vi "TA Binding Data to String.vi"(8 "error in (no error)":errorcluster, 10 "TA Binding Data":T1, 11 "Motions in":refnum<class "Motions.lvclass">) -> (0 "error out":errorcluster, 2 "String":string, 3 "Motions out":refnum<class "Motions.lvclass">)   [LabVIEW 2016, in "Hardware.lvlib" / "Motions.lvlib" / "Motions.lvclass"]
uses:
  <userlib>/Common Components/Hardware/Abstract System/Motions/Motions/Motions.lvclass
  <userlib>/Common Components/Hardware/Abstract System/Motions/Motions/TA Binding Data.ctl
  <userlib>/Common Components/Hardware/Abstract System/Motions/Motions/Motions.lvclass/Motions.ctl
  <userlib>/Common Components/Hardware/Abstract Hardware/Hardware.lvclass/Hardware.ctl
  <userlib>/Common Components/Hardware/Abstract Hardware/Read Label.vi
  <userlib>/Common Components/Hardware/Motor/Motor/Motor.lvclass
  C:/Program Files (x86)/National Instruments/LabVIEW 2016/user.lib/Common Components/Hardware/Abstract Hardware/Hardware.lvclass
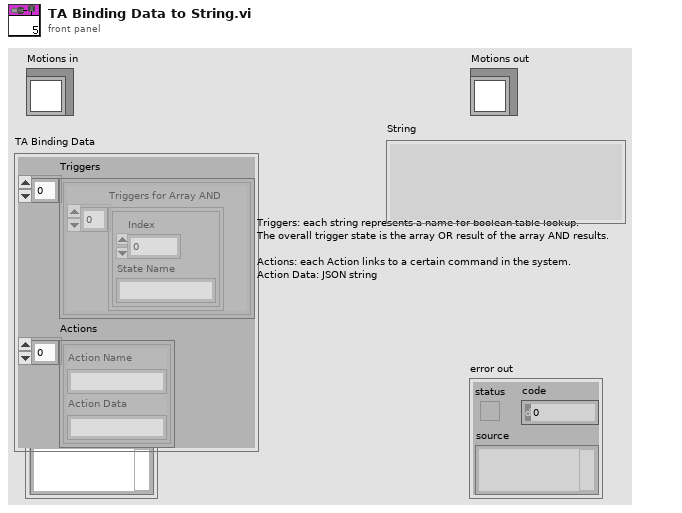
[diagram p1: front panel]
types:
  T1 = typedef "Hardware.lvlib/Motions.lvlib/Motions.lvclass/TA Binding Data.ctl" = cluster{"Triggers":cluster{"Triggers for Array AND":cluster{"Index":u8, "State Name":string}[]}[], "Actions":cluster{"Action Name":string, "Action Data":string}[]}
  T2 = cluster{"Triggers for Array AND":cluster{"Index":u8, "State Name":string}[]}[]
  T3 = cluster{"Action Name":string, "Action Data":string}[]
  T4 = cluster{"Action Name":string, "JSON info":cluster{"path":string, "data type":enum16{"INT", "DBL", "BOOL", "String"}}[], "String Format":string}[]
  T5 = cluster{"path":string, "data type":enum16{"INT", "DBL", "BOOL", "String"}}[]
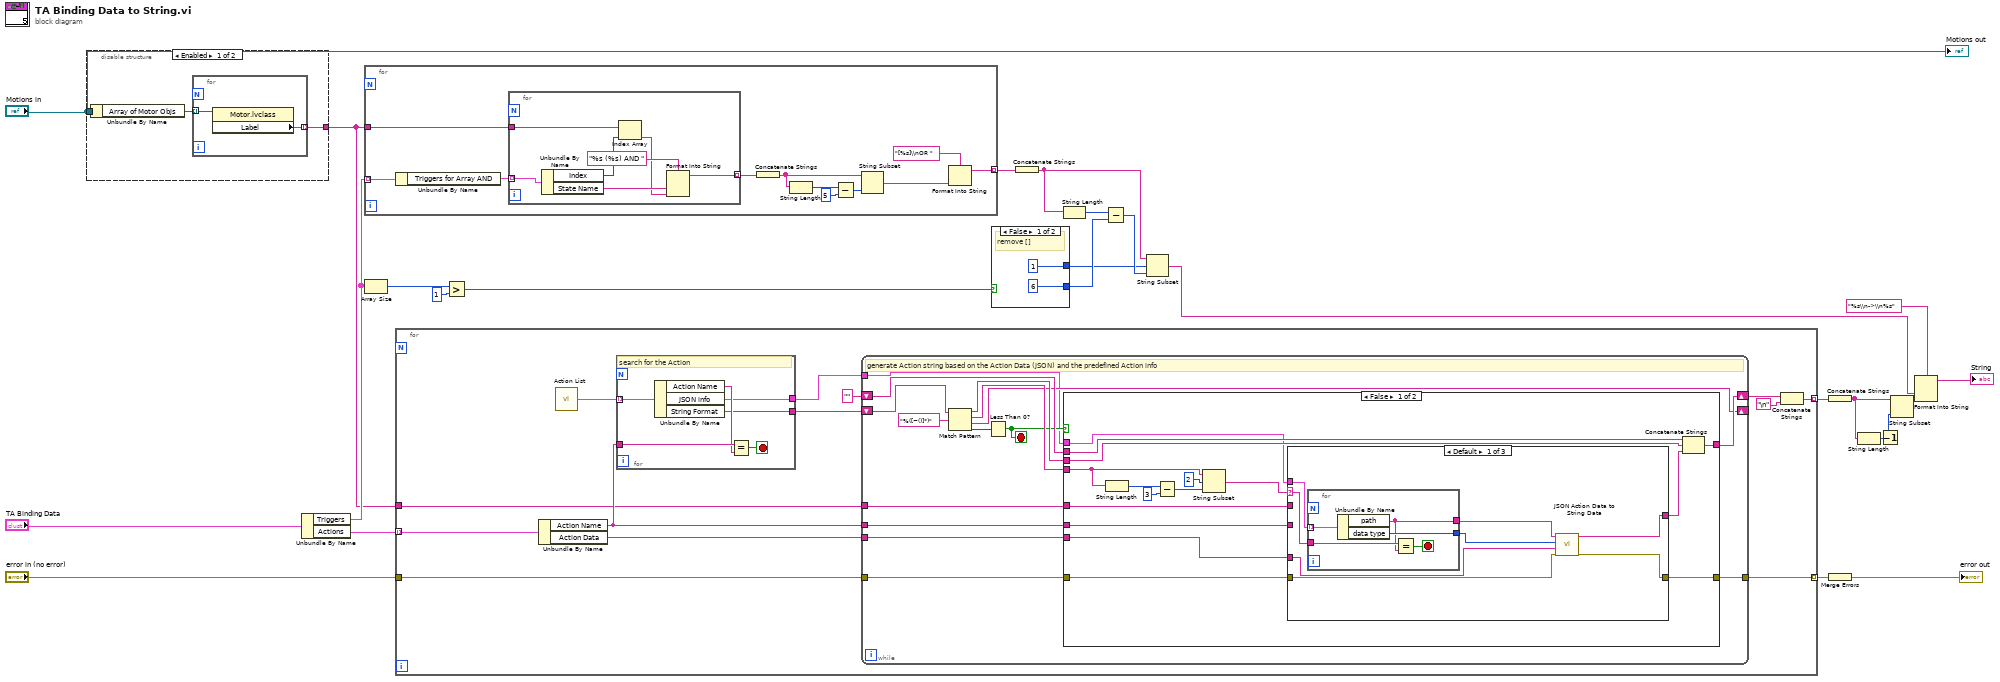
[diagram p0: block diagram]
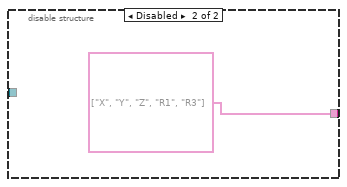
[diagram p2: hidden frame]
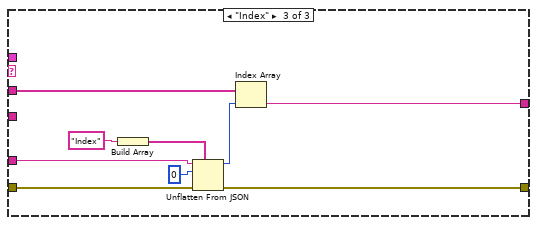
[diagram p4: hidden frame]
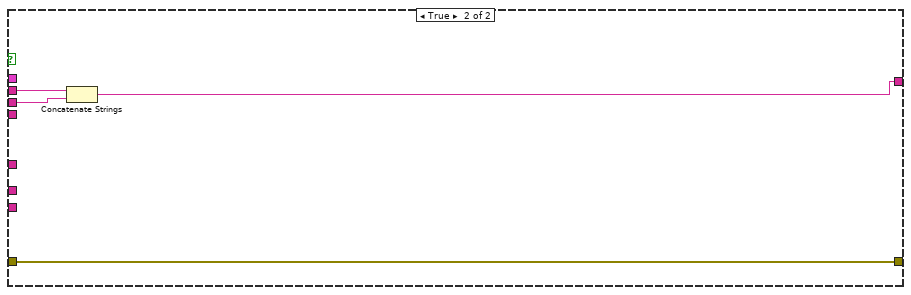
[diagram p5: hidden frame]
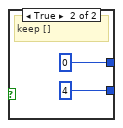
[diagram p6: hidden frame]
diagram:
  n1 = disable-structure shown="Enabled" {
    disable-tunnel: "Motions in" -> [w28 _]
    disable-tunnel: [w26 string[] ["X", "Y", "Z", "R1", "R3"]] -> w9
    frame Enabled {
      n2 = Unbundle By Name(w28) -> ("Array of Motor Objs"=w27:refnum<class "Motor.lvclass">[])
      n3 = for {
        tunnel: w27 -> [w30] mode=indexing
        tunnel: [w29] -> w26 mode=indexing
        n4 = property class="Motor.lvclass"(reference=w30) -> ("Label"=w29:string)  [unwired: 1 in, 2 out]
      }
    }
    frame Disabled {
    }
  }
  n5 = Unbundle By Name("TA Binding Data") -> ("Triggers"=w18:T2, "Actions"=w10:T3)
  n6 = for {
    tunnel: w18 -> [w42] mode=indexing
    tunnel: w9 -> [w40]
    tunnel: [w34] -> w19 mode=indexing
    n7 = Unbundle By Name(w42) -> ("Triggers for Array AND"=w41:cluster{"Index":u8, "State Name":string}[])
    n8 = for {
      tunnel: w41 -> [w49] mode=indexing
      tunnel: w40 -> [w46]
      tunnel: [w43] -> w39 mode=indexing
      n9 = Unbundle By Name(w49) -> ("Index"=w45:u8, "State Name"=w47:string)
      n10 = Index Array(array=w46, index=w45) -> (element=w44:string)
      n11 = Format Into String(format string="%s (%s) AND ", w47, w44) -> (resulting string=w43:string)  [unwired: 2 in, 1 out]
    }
    n12 = Concatenate Strings(w39) -> (w38:string)
    n13 = String Length(string=w38) -> (length=w37:i32)
    n14 = Subtract(x=w37, y=5) -> (x-y=w35:i32)
    n15 = String Subset(string=w38, length (rest)=w35) -> (substring=w32:string)  [unwired: 1 in]
    n16 = Format Into String(format string="[%s]\\nOR ", w32) -> (resulting string=w34:string)  [unwired: 2 in, 1 out]
  }
  n17 = Array Size(array=w18) -> (size(s)=w17:i32)
  n18 = for {
    tunnel: w10 -> [w62] mode=indexing
    tunnel: [w52] -> w8 mode=indexing
    tunnel: w9 -> [w55]
    tunnel: "error in (no error)" -> [w51]
    tunnel: [w50] -> w6 mode=indexing
    n19 = Unbundle By Name(w62) -> ("Action Name"=w58:string, "Action Data"=w56:string)
    n20 = call <userlib>:"Action List.vi"() -> ("Action List"=w61:T4)
    n21 = for {
      tunnel: w61 -> [w127] mode=indexing
      tunnel: w58 -> [w126]
      tunnel: [w123] -> w54
      tunnel: [w122] -> w60
      stop <- w124 stop-if-true
      # "search for the Action"
      n22 = Unbundle By Name(w127) -> ("Action Name"=w125:string, "JSON info"=w123:T5, "String Format"=w122:string)
      n23 = Equal?(x=w126, y=w125) -> (x = y?=w124:bool)
    }
    n24 = while {
      shift-right: [w72] -> w57
      shift-left: "" -> [w74]
      tunnel: w58 -> [w70]
      shift-right: [w69] -> _
      shift-left: w60 -> [w77]
      tunnel: w56 -> [w67]
      tunnel: w55 -> [w66]
      tunnel: w54 -> [w65]
      tunnel: w51 -> [w64]
      tunnel: [w63] -> w50
      stop <- w68 stop-if-true
      # "generate Action string based on the Action Data (JSON) and the predefined Action info"
      n25 = Match Pattern(string=w77, regular expression="%([~()]*)") -> (before substring=w73:string, match substring=w71:string, after substring=w69:string, offset past match=w75:i32)  [unwired: 1 in]
      n26 = Less Than 0?(x=w75) -> (x < 0?=w68:bool)
      n27 = case shown="False" w68 {
        tunnel: w74 -> [w93 w121]
        tunnel: w73 -> [w92 w120]
        tunnel: [w91 w119] -> w72
        tunnel: w71 -> [w89 _]
        tunnel: w70 -> [w84 _]
        tunnel: w67 -> [w82 _]
        tunnel: w66 -> [w81 _]
        tunnel: w65 -> [w80 _]
        tunnel: w64 -> [w79 w118]
        tunnel: [w78 w118] -> w63
        frame False {
          n28 = String Length(string=w89) -> (length=w88:i32)
          n29 = Subtract(x=w88, y=3) -> (x-y=w86:i32)
          n30 = String Subset(string=w89, offset (0)=2, length (rest)=w86) -> (substring=w85:string)
          n31 = case shown="Default" w85 {
            selector: w85 -> [w100 _ _]
            tunnel: w84 -> [_ w108 _]
            tunnel: [w96 w108 w111] -> w83
            tunnel: w82 -> [w98 _ w116]
            tunnel: w81 -> [_ _ w113]
            tunnel: w80 -> [w101 _ _]
            tunnel: w79 -> [w95 w107 w110]
            tunnel: [w94 w107 w109] -> w78
            frame Default {
              n32 = for {
                tunnel: w101 -> [w106] mode=indexing
                tunnel: w100 -> [w105]
                tunnel: [w103] -> w99
                tunnel: [w102] -> w97
                stop <- w104 stop-if-true
                n33 = Unbundle By Name(w106) -> ("path"=w102:string, "data type"=w103:enum16{"INT", "DBL", "BOOL", "String"})
                n34 = Equal?(x=w105, y=w102) -> (x = y?=w104:bool)
              }
              n35 = call <userlib>:"JSON Action Data to String Data.vi"("error in (no error)"=w95, "Action Data (JSON)"=w98, "data type"=w99, "path"=w97) -> ("error out"=w94:errorcluster, "String"=w96:string)  [unwired: 6 in]
            }
            frame "Action Name" {
            }
            frame "Index" {
              n36 = Build Array("Index") -> (w117:string[])
              n37 = Unflatten From JSON(path=w117, JSON string=w116, type and defaults=0, error in (no error)=w110) -> (value=w112:i32, error out=w109:errorcluster)  [unwired: 3 in]
              n38 = Index Array(array=w113, index=w112) -> (element=w111:string)
            }
          }
          n39 = Concatenate Strings(w93, w92, w83) -> (w91:string)
        }
        frame True {
          n40 = Concatenate Strings(w121, w120) -> (w119:string)
        }
      }
    }
    n41 = Concatenate Strings(w57, "\n") -> (w52:string)
  }
  n42 = Greater?(x=w17, y=1) -> (0:w15:bool)
  n43 = case shown="False" w15 {
    tunnel: [6 ("y") 4 ("y")] -> w21
    tunnel: [1 ("y") 0 ("y")] -> w14
    frame False {
      # "remove []"
    }
    frame True {
      # "keep []"
    }
  }
  n44 = Concatenate Strings(w19) -> (w23:string)
  n45 = String Length(string=w23) -> (length=w22:i32)
  n46 = Subtract(x=w22, y=w21) -> (x-y=w20:i32)
  n47 = String Subset(string=w23, offset (0)=w14, length (rest)=w20) -> (substring=w12:string)
  n48 = Concatenate Strings(w8) -> (w2:string)
  n49 = Merge Errors(w6) -> (→"error out":errorcluster)
  n50 = String Length(string=w2) -> (length=w3:i32)
  n51 = Decrement(x=w3) -> (x-1=w1:i32)
  n52 = String Subset(string=w2, length (rest)=w1) -> (substring=w4:string)  [unwired: 1 in]
  n53 = Format Into String(format string="%s\\n->\\n%s", w12, w4) -> (resulting string=→"String":string)  [unwired: 2 in, 1 out]
  "Motions out" <- "Motions in"
